vi "xiCam - SetParam_Int32.vi"(6 "Int32_Value":i32, 7 "PRM":T1, 8 "error in (no error)":errorcluster, 11 "xiCam In":refnum<k24>) -> (0 "error out":errorcluster, 3 "xiCam Out":refnum<k24>)   [LabVIEW 2018]
doc: "This function configures the device.\n\n<b>void SetParam(string prm, int val)</b>\nstring prm : Parameter name string. Use class PRM to set parameters.\nint val : Integer value to be set."
uses:
  C:/XIMEA/API/x64/xiApi.NETX64.dll
  PRM/PRM/PRM_v2.ctl
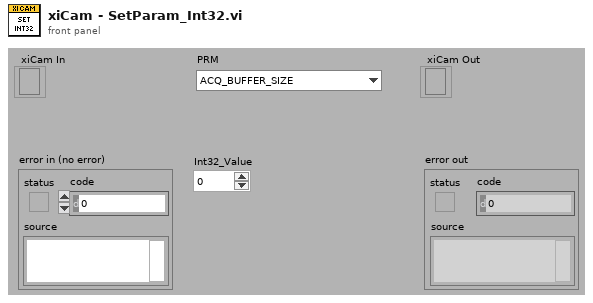
[diagram p1: front panel]
types:
  T1 = typedef "PRM_v2.ctl" = enum16{"ACQ_BUFFER_SIZE", "ACQ_FRAME_BURST_COUNT", "ACQ_TIMING_MODE", "ACQ_TRANSPORT_BUFFER_SIZE", "AE_MAX_LIMIT", "AEAG", "AEAG_LEVEL", "API_VERSION", "AG_MAX_LIMIT", "APPLY_CMS", "AUTO_BANDWIDTH_CALCULATION", "AUTO_WB", "AVAILABLE_BANDWIDTH", "AVAILABLE_BANDWIDTH_MAX", "AVAILABLE_BANDWIDTH_MIN", "BPC", "BUFFER_POLICY", "BUFFERS_QUEUE_SIZE", "CC_MATRIX_00", "CC_MATRIX_01", "CC_MATRIX_02", "CC_MATRIX_03", "CC_MATRIX_10", "CC_MATRIX_11", "CC_MATRIX_12", "CC_MATRIX_13", "CC_MATRIX_20", "CC_MATRIX_21", "CC_MATRIX_22", "CC_MATRIX_23", "CC_MATRIX_30", "CC_MATRIX_31", "CC_MATRIX_32", "CC_MATRIX_33", "CHIP_TEMP", "CMS", "COLOR_FILTER_ARRAY", "COOLING", "DEBOUNCE_EN", "DEBOUNCE_POL", "DEBOUNCE_T0", "DEBOUNCE_T1", "DEBUG_LEVEL", "DEFAULT_CC_MATRIX", "DEVICE_INSTANCE_PATH", "DEVICE_MODEL_ID", "DEVICE_NAME", "DEVICE_SN", "DEVICE_TYPE", "DEVICE_USER_ID", "DOWNSAMPLING", "DOWNSAMPLING_MAX", "DOWNSAMPLING_MIN", "DOWNSAMPLING_TYPE", "DRV_VERSION", "EXP_PRIORITY", "EXPOSURE", "EXPOSURE_DIRECT_UPDATE", "EXPOSURE_MAX", "EXPOSURE_MIN", "FFS_FILE_NAME", "FPGA1_VERSION", "FRAMERATE", "FRAMERATE_MAX", "FRAMERATE_MIN", "FREE_FFS_SIZE", "GAIN", "GAIN_DIRECT_UPDATE", "GAIN_MAX", "GAIN_MIN", "GAMMAC", "GAMMAY", "GPI_LEVEL", "GPI_MODE", "GPI_SELECTOR", "GPI_SELECTOR_MAX", "GPI_SELECTOR_MIN", "GPO_MODE", "GPO_SELECTOR", "GPO_SELECTOR_MAX", "GPO_SELECTOR_MIN", "HDR", "HDR_T1", "HDR_T2", "HEIGHT", "HEIGHT_MAX", "HEIGHT_MIN", "HOUSE_TEMP", "IMAGE_DATA_FORMAT", "IMAGE_IS_COLOR", "INPUT_CMS_PROFILE", "IS_COOLED", "IS_DEVICE_EXIST", "KNEEPOINT1", "KNEEPOINT2", "LED_MODE", "LED_SELECTOR", "LED_SELECTOR_MAX", "LED_SELECTOR_MIN", "LIMIT_BANDWIDTH", "LIMIT_BANDWIDTH_MAX", "LIMIT_BANDWIDTH_MIN", "LUT_EN", "LUT_INDEX", "LUT_INDEX_MAX", "LUT_INDEX_MIN", "LUT_VALUE", "LUT_VALUE_MAX", "LUT_VALUE_MIN", "MANUAL_WB", "MCU1_VERSION", "MCU2_VERSION", "OFFSET_X", "OFFSET_X_MAX", "OFFSET_X_MIN", "OFFSET_Y", "OFFSET_Y_MAX", "OFFSET_Y_MIN", "OUTPUT_CMS_PROFILE", "OUTPUT_DATA_BIT_DEPTH", "OUTPUT_DATA_PACKING", "READ_FILE_FFS", "RECENT_FRAME", "SENSOR_DATA_BIT_DEPTH", "SENSOR_MODE", "SENSOR_TAPS", "SHARPNESS", "SHUTTER_TYPE", "TARGET_TEMP", "TRG_DELAY", "TRG_SELECTOR", "TRG_SOFTWARE", "TRG_SOURCE", "USED_FFS_SIZE", "WB_KB", "WB_KG", "WB_KR", "WIDTH", "WIDTH_MAX", "WIDTH_MIN", "WRITE_FILE_FFS", "ACQ_BUFFER_SIZE_UNIT", "ACQ_TRANSPORT_BUFFER_COMMIT", "AEAG_ROI_HEIGHT", "AEAG_ROI_OFFSET_X", "AEAG_ROU_OFFSET_Y", "AEAG_ROI_WIDTH", "API_CONTEXT_LIST", "BINNING_HORIZONTAL", "BINNING_SELECTOR", "BINNING_VERTICAL", "COLUMN_FPN_CORRECTION", "COUNTER_SELECTOR", "COUNTER_VALUE", "DECIMATION_HORIZONTAL", "DECIMATION_SELECTOR", "DECIMATION_VERTICAL", "DEVICE_ID", "DEVICE_LOCATION_PATH", "DEVICE_MANIFEST", "DEVICE_RESET", "DEVICE_SENS_SN", "EXPOSURE_BURST_COUNT", "FFS_ACCESS_KEY", "GAIN_SELECTOR", "HW_REVISION", "IMAGE_BLACK_LEVEL", "IMAGE_DATA_BIT_DEPTH", "IMAGE_DATA_FORMAT_RGB32_ALPHA", "IMAGE_PAYLOAD_SIZE", "LENS_APERTURE_VALUE", "LENS_FEATURE", "LENS_FEATURE_SELECTOR", "LENS_FOCAL_LENGTH", "LENS_FOCUS_DISTANCE", "LENS_FOCUS_MOVE", "LENS_FOCUS_MOVEMENT_VALUE", "LENS_MODE", "OUTPUT_DATA_PACKING_TYPE", "SENSOR_CLOCK_FREQ_HZ", "SENSOR_CLOCK_FREQ_INDEX", "SENSOR_FEATURE_SELECTOR", "SENSOR_FEATURE_VALUE", "SENSOR_OUTPUT_CHANNEL_COUNT", "TRANSPORT_PIXEL_FORMAT", "TS_RST_MODE", "TS_RST_SOURCE"}
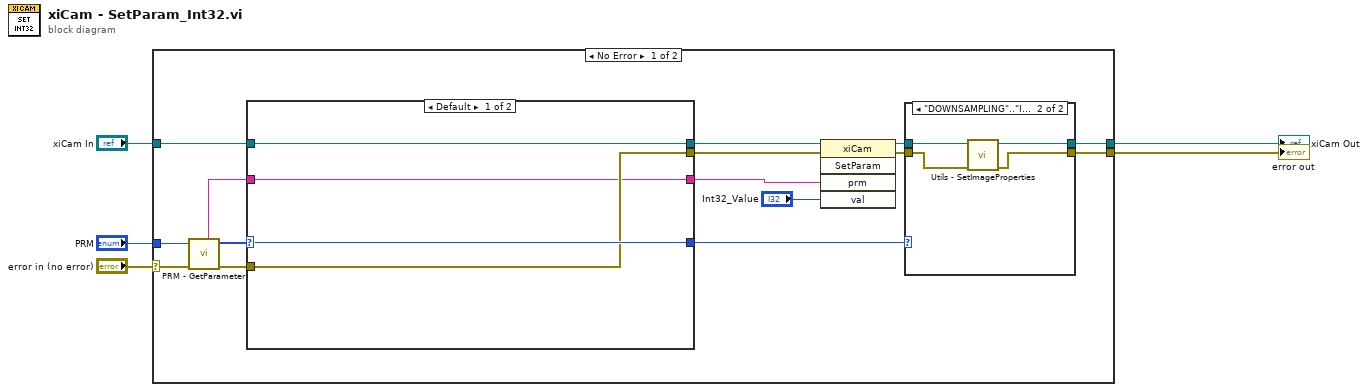
[diagram p0: block diagram]
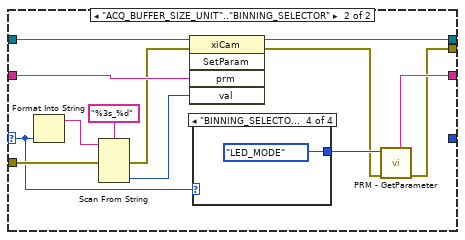
[diagram p3: hidden frame]
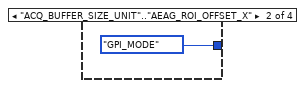
[diagram p5: hidden frame]
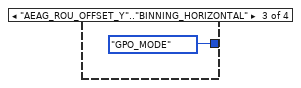
[diagram p6: hidden frame]
diagram:
  n1 = case shown="No Error" "error in (no error)" {
    selector: "error in (no error)" -> [w20 w47]
    tunnel: "xiCam In" -> [w18 w48]
    tunnel: [w7 w48] -> w3
    tunnel: [w6 w47] -> w2
    tunnel: "PRM" -> [w16 _]
    frame No Error {
      n2 = call "PRM - GetParameter.vi"("error in (no error)"=w20, "PRM"=w16) -> ("error out"=w17:errorcluster, "PRM OUT"=w14:T1, "ParameterString"=w19:string)  [unwired: 7 in]
      n3 = case shown="Default" w14 {
        selector: w14 -> [w30 w31]
        tunnel: w19 -> [w27 w42]
        tunnel: w18 -> [w29 w43]
        tunnel: w17 -> [w28 w38]
        tunnel: [w30 _] -> w10
        tunnel: [w29 w41] -> w15
        tunnel: [w27 w33] -> w13
        tunnel: [w28 w32] -> w12
        frame Default {
        }
        frame "ACQ_BUFFER_SIZE_UNIT".."BINNING_SELECTOR" {
          n4 = Format Into String(w31) -> (resulting string=w40:string)  [unwired: 3 in, 1 out]
          n5 = Scan From String(format string="%3s_%d", input string=w40, error in=w38) -> (error out=w35:errorcluster, output 2=w37:i32)  [unwired: 4 in, 2 out]
          n6 = invoke class="xiCam" method="SetParam"(reference=w43, error in=w35, "prm"=w42, "val"=w37) -> (reference out=w41:refnum<k24>, error out=w34:errorcluster)  [unwired: 1 in, 3 out]
          n7 = case shown="\"BINNING_SELECTOR\"" w31 {
            tunnel: [_ PRM_v2."GPI_MODE" ("PRM") PRM_v2."GPO_MODE" ("PRM") PRM_v2."LED_MODE" ("PRM")] -> w36
            frame Default {
            }
            frame "ACQ_BUFFER_SIZE_UNIT".."AEAG_ROI_OFFSET_X" {
            }
            frame "AEAG_ROU_OFFSET_Y".."BINNING_HORIZONTAL" {
            }
            frame "BINNING_SELECTOR" {
            }
          }
          n8 = call "PRM - GetParameter.vi"("error in (no error)"=w34, "PRM"=w36) -> ("error out"=w32:errorcluster, "ParameterString"=w33:string)  [unwired: 7 in, 1 out]
        }
      }
      n9 = invoke class="xiCam" method="SetParam"(reference=w15, error in=w12, "prm"=w13, "val"="Int32_Value") -> (reference out=w8:refnum<k24>, error out=w9:errorcluster)  [unwired: 1 in, 3 out]
      n10 = case shown="\"DOWNSAMPLING\"..\"IMAGE_DATA_FORMAT\", \"WIDTH\"" w10 {
        tunnel: w9 -> [w21 w25]
        tunnel: w8 -> [w22 w26]
        tunnel: [w22 w24] -> w7
        tunnel: [w21 w23] -> w6
        frame Default {
        }
        frame "DOWNSAMPLING".."IMAGE_DATA_FORMAT", "WIDTH" {
          n11 = call "Utils - SetImageProperties.vi"("error in (no error)"=w25, "xiCam In"=w26) -> ("error out"=w23:errorcluster, "xiCam Out"=w24:refnum<k24>)  [unwired: 8 in]
        }
      }
    }
    frame Error {
    }
  }
  "error out" <- w2
  "xiCam Out" <- w3
